vi "Terminal-Main-LoadingUnit.vi"(4 "ErrorQRef":refnum<queue>, 5 "ModbusNResRef":refnum<notifier>, 6 "ModbusMsgQRef":refnum<queue>, 7 "ModbusNReqRef":refnum<notifier>, 8 "error in (no error)":errorcluster caption="错误输入（无错误）", 11 "LoadingUnitNRef":refnum<notifier>) -> (0 "error out":errorcluster caption="错误输出")   [LabVIEW 2014]
panel:
  out "Loading Unit is running":bool
  out "LoadingUnit开始通知器":refnum<notifier>
  out "LoadingUnit开始响应器":refnum<notifier>
  out "LoadingUnit停止通知器":refnum<notifier>
  out "LoadingUnit停止响应器":refnum<notifier>
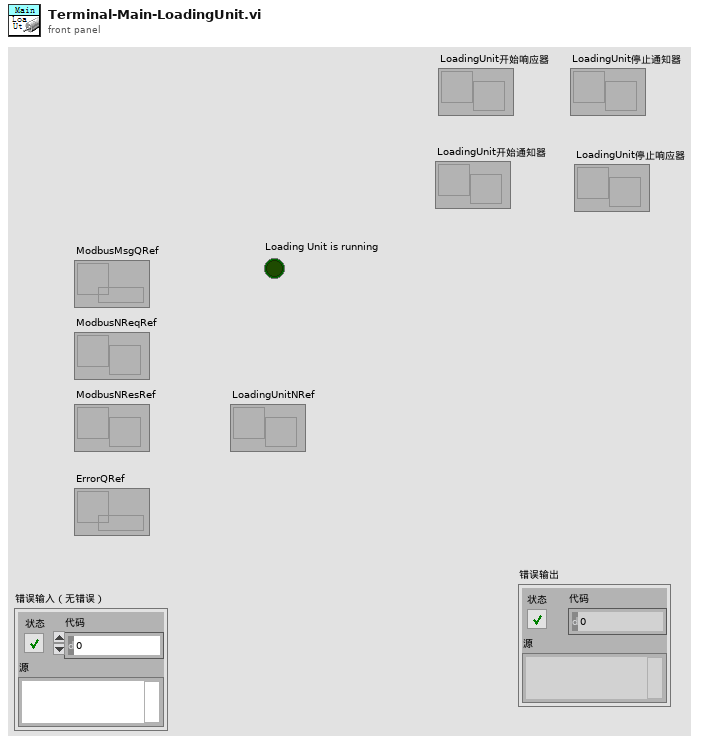
[diagram p1: front panel]
types:
  T1 = cluster{"Transaction ID":u16, "Unit ID":u8, "Starting Address":u16, "Quantity":u16}
  T2 = cluster{"Transaction ID":u16, "Unit ID":u8, "Address":u16, "Register":u16}
  T3 = cluster{"Transaction ID":u16, "Unit ID":u8, "Starting Address":u16, "Registers":u16[]}
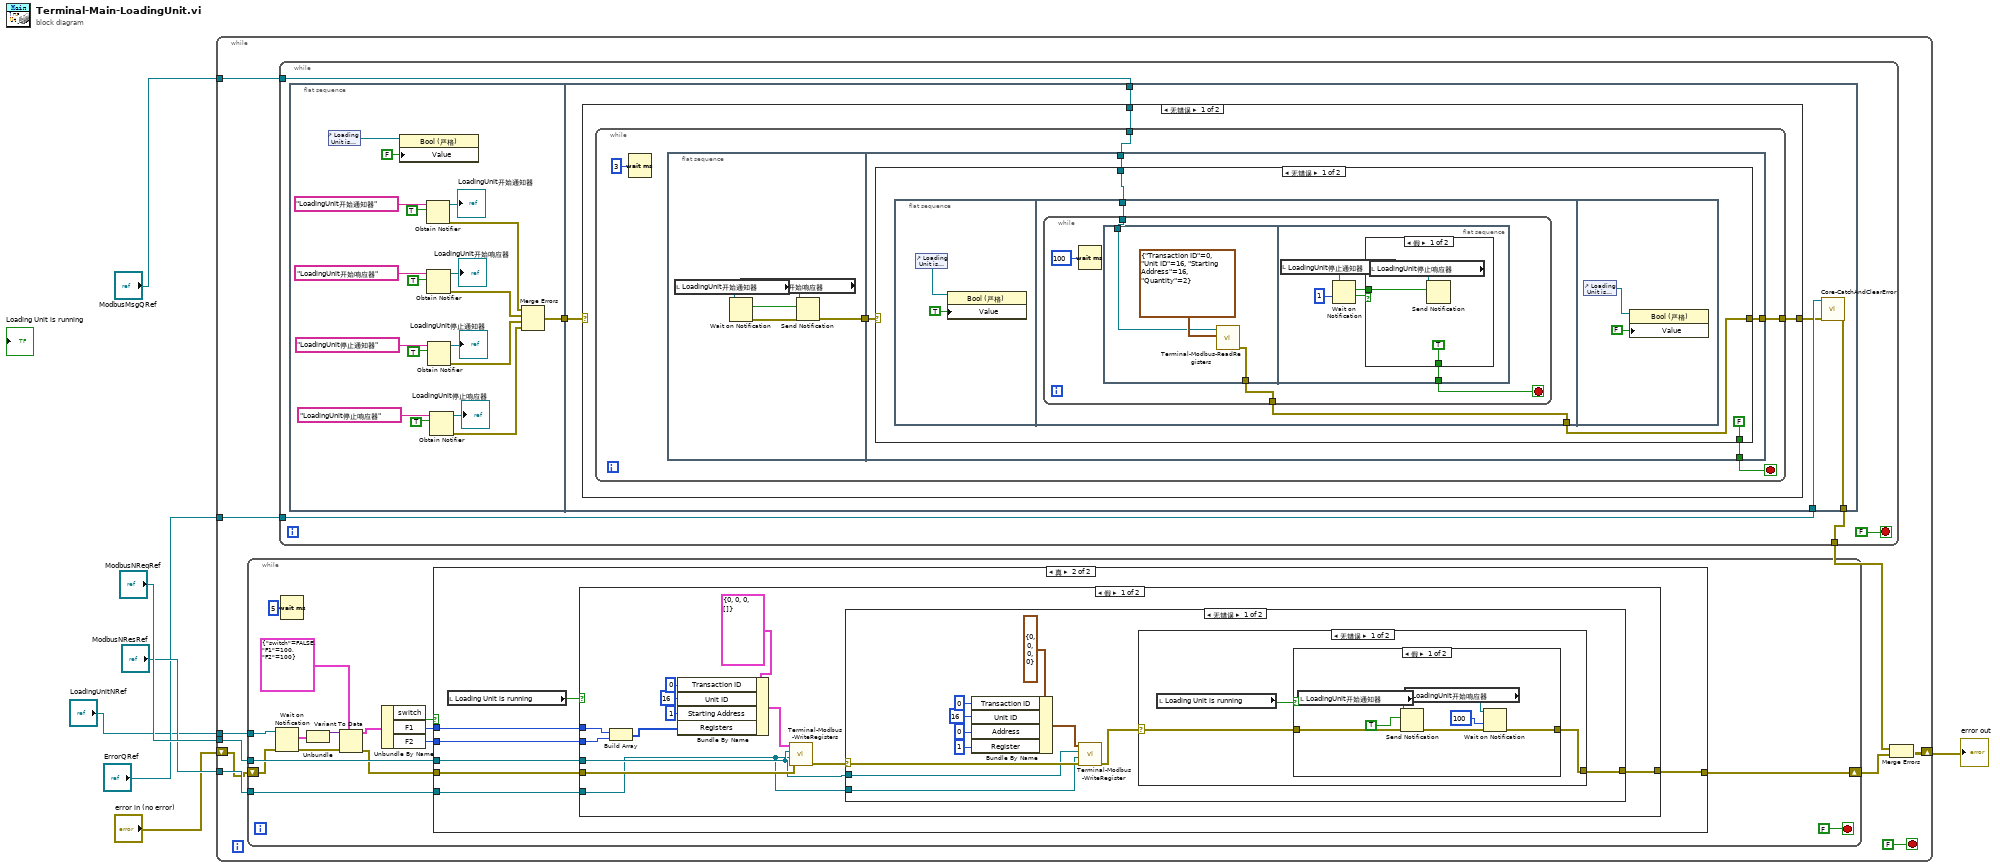
[diagram p0: block diagram]
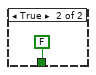
[diagram p2: hidden frame]
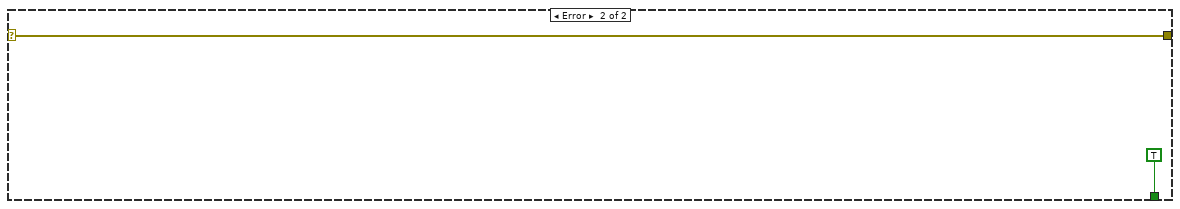
[diagram p3: hidden frame]
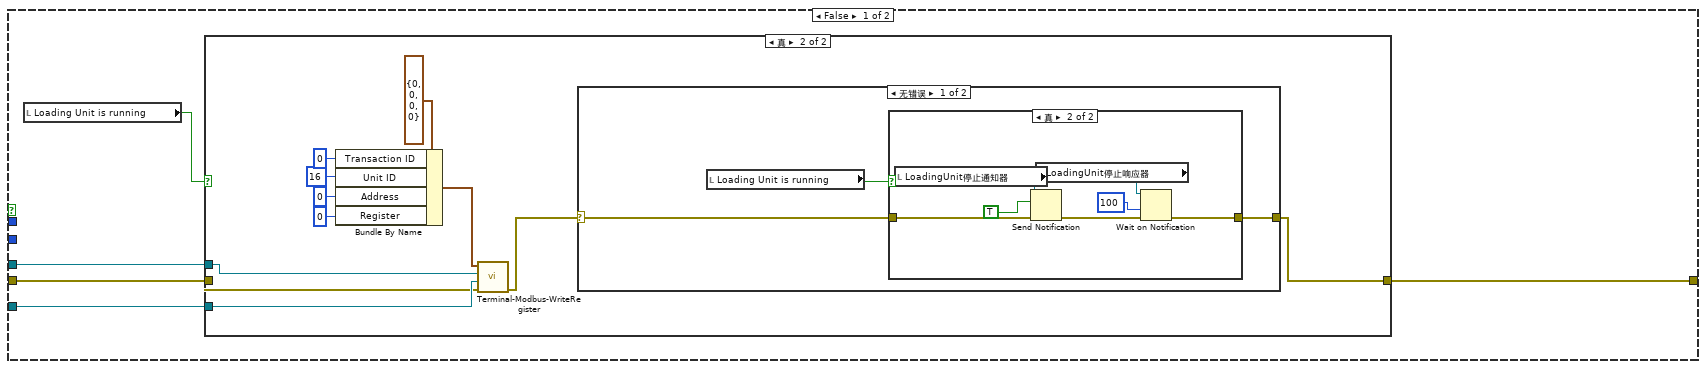
[diagram p5: hidden frame]
diagram:
  n1 = while {
    tunnel: "ModbusMsgQRef" -> [w17]
    tunnel: "ModbusNReqRef" -> [w16]
    tunnel: "ModbusNResRef" -> [w15]
    tunnel: "ErrorQRef" -> [w13]
    shift-right: [w12] -> w2
    shift-left: "error in (no error)" -> [w14]
    tunnel: "LoadingUnitNRef" -> [w8]
    stop <- FALSE stop-if-true
    n2 = while {
      tunnel: w16 -> [w106]
      tunnel: w15 -> [w105]
      shift-right: [w104] -> w11
      shift-left: w14 -> [w100]
      tunnel: w8 -> [w101]
      stop <- FALSE stop-if-true
      n3 = Wait on Notification(notifier=w101, error in (no error)=w100) -> (notification=w99:cluster{variant, string}, error out=w94:errorcluster)  [unwired: 2 in, 2 out]
      n4 = Wait (ms)(milliseconds to wait=u32 5 ("等待时间（毫秒）")) -> ()  [unwired: 1 out]
      n5 = Unbundle(w99) -> (w98:variant)  [unwired: 1 out]
      n6 = Variant To Data(error in=w94, type=cluster{"switch":bool, "F1":u16, "F2":u16} {"switch"=FALSE, "F1"=100, "F2"=100}, Variant=w98) -> (data=w97:cluster{"switch":bool, "F1":u16, "F2":u16}, error out=w93:errorcluster)
      n7 = Unbundle By Name(w97) -> ("switch"=w96:bool, "F1"=w95:u16, "F2"=w91:u16)
      n8 = case shown="真" w96 {
        tunnel: w106 -> [w111 w140]
        tunnel: w105 -> [w110 w141]
        tunnel: w93 -> [w109 w142]
        tunnel: [w108 w139] -> w104
        tunnel: w95 -> [_ w138]
        tunnel: w91 -> [_ w136]
        frame False {
          n9 = local read "Loading Unit is running"() -> (w107:bool)
          n10 = case shown="真" w107 {
            tunnel: w111 -> [_ w122]
            tunnel: w110 -> [_ w121]
            tunnel: w109 -> [w112 w120]
            tunnel: [w112 w119] -> w108
            frame False {
            }
            frame True {
              n11 = Bundle By Name(cluster=T2 {"Transaction ID"=0, "Unit ID"=0, "Address"=0, "Register"=0} ("簇"), "Transaction ID"=u16 0, "Unit ID"=u8 16, "Address"=u16 0, "Register"=u16 0) -> (w114:T2)
              n12 = call "Terminal-Modbus-WriteRegister.vi"("error in (no error)"=w120, "ModbusNResRef"=w121, "ModbusNReqRef"=w122, "簇"=w114) -> ("error out"=w123:errorcluster)  [unwired: 7 in]
              n13 = case shown="无错误" w123 {
                selector: w123 -> [w125 w135]
                tunnel: [w124 w135] -> w119
                frame No Error {
                  n14 = local read "Loading Unit is running"() -> (w126:bool)
                  n15 = case shown="真" w126 {
                    tunnel: [w127 w129] -> w124
                    tunnel: w125 -> [w127 w128]
                    frame False {
                    }
                    frame True {
                      n16 = local read "LoadingUnit停止通知器"() -> (w134:refnum<notifier>)
                      n17 = Send Notification(notification=TRUE ("通知"), notifier=w134, error in (no error)=w128) -> (error out=w132:errorcluster)  [unwired: 1 out]
                      n18 = local read "LoadingUnit停止响应器"() -> (w131:refnum<notifier>)
                      n19 = Wait on Notification(notifier=w131, timeout in ms (-1)=100 ("超时毫秒(-1)"), error in (no error)=w132) -> (error out=w129:errorcluster)  [unwired: 1 in, 3 out]
                    }
                  }
                }
                frame Error {
                }
              }
            }
          }
        }
        frame True {
          n20 = local read "Loading Unit is running"() -> (w137:bool)
          n21 = case shown="假" w137 {
            tunnel: w142 -> [w154 w180]
            tunnel: w141 -> [w143 _]
            tunnel: w140 -> [w144 _]
            tunnel: [w153 w180] -> w139
            tunnel: w138 -> [w152 _]
            tunnel: w136 -> [w151 _]
            frame False {
              n22 = Build Array(w152, w151) -> (w145:u16[])
              n23 = Bundle By Name(cluster=T3 {"Transaction ID"=0, "Unit ID"=0, "Starting Address"=0, "Registers"=[]} ("簇"), "Transaction ID"=u16 0, "Unit ID"=u8 16, "Starting Address"=u16 1 ("Address"), "Registers"=w145) -> (w147:T3)
              n24 = call "Terminal-Modbus-WriteRegisters.vi"("error in (no error)"=w154, "ModbusNResRef"=w143, "ModbusNReqRef"=w144, "簇"=w147) -> ("error out"=w155:errorcluster)  [unwired: 7 in]
              n25 = case shown="无错误" w155 {
                selector: w155 -> [w165 w179]
                tunnel: w144 -> [w164 _]
                tunnel: w143 -> [w163 _]
                tunnel: [w162 w179] -> w153
                frame No Error {
                  n26 = Bundle By Name(cluster=T2 {"Transaction ID"=0, "Unit ID"=0, "Address"=0, "Register"=0} ("簇"), "Transaction ID"=u16 0, "Unit ID"=u8 16, "Address"=u16 0, "Register"=u16 1) -> (w157:T2)
                  n27 = call "Terminal-Modbus-WriteRegister.vi"("error in (no error)"=w165, "ModbusNResRef"=w163, "ModbusNReqRef"=w164, "簇"=w157) -> ("error out"=w166:errorcluster)  [unwired: 7 in]
                  n28 = case shown="无错误" w166 {
                    selector: w166 -> [w168 w178]
                    tunnel: [w167 w178] -> w162
                    frame No Error {
                      n29 = local read "Loading Unit is running"() -> (w169:bool)
                      n30 = case shown="假" w169 {
                        tunnel: [w171 w177] -> w167
                        tunnel: w168 -> [w170 w177]
                        frame False {
                          n31 = local read "LoadingUnit开始通知器"() -> (w176:refnum<notifier>)
                          n32 = Send Notification(notification=TRUE ("通知"), notifier=w176, error in (no error)=w170) -> (error out=w174:errorcluster)  [unwired: 1 out]
                          n33 = local read "LoadingUnit开始响应器"() -> (w173:refnum<notifier>)
                          n34 = Wait on Notification(notifier=w173, timeout in ms (-1)=100 ("超时毫秒(-1)"), error in (no error)=w174) -> (error out=w171:errorcluster)  [unwired: 1 in, 3 out]
                        }
                        frame True {
                        }
                      }
                    }
                    frame Error {
                    }
                  }
                }
                frame Error {
                }
              }
            }
            frame True {
            }
          }
        }
      }
    }
    n35 = while {
      tunnel: w17 -> [w21]
      tunnel: w13 -> [w20]
      tunnel: [w18] -> w10
      stop <- FALSE stop-if-true
      n36 = flat-sequence {
        tunnel: [w24] -> w22
        tunnel: w22 -> [w46]
        tunnel: w20 -> [w45]
        tunnel: [w43] -> w18
        tunnel: w21 -> [w42]
        frame #0 {
          n37 = control-ref of="Loading Unit is running"() -> (w23:refnum<vi>)
          n38 = property class="Bool (严格)"(reference=w23, "Value"=FALSE ("值")) -> ()  [unwired: 1 in, 2 out]
          n39 = Obtain Notifier(name (unnamed)="LoadingUnit开始通知器" ("名称（未命名）"), notification data type=TRUE) -> (notifier out=→"LoadingUnit开始通知器":refnum<notifier>, error out=w28:errorcluster)  [unwired: 2 in, 1 out]
          n40 = Obtain Notifier(name (unnamed)="LoadingUnit开始响应器" ("名称（未命名）"), notification data type=TRUE) -> (notifier out=→"LoadingUnit开始响应器":refnum<notifier>, error out=w27:errorcluster)  [unwired: 2 in, 1 out]
          n41 = Obtain Notifier(name (unnamed)="LoadingUnit停止通知器" ("名称（未命名）"), notification data type=TRUE) -> (notifier out=→"LoadingUnit停止通知器":refnum<notifier>, error out=w26:errorcluster)  [unwired: 2 in, 1 out]
          n42 = Obtain Notifier(name (unnamed)="LoadingUnit停止响应器" ("名称（未命名）"), notification data type=TRUE) -> (notifier out=→"LoadingUnit停止响应器":refnum<notifier>, error out=w25:errorcluster)  [unwired: 2 in, 1 out]
          n43 = Merge Errors(w28, w27, w26, w25) -> (w24:errorcluster)
        }
        frame #1 {
          n44 = case shown="无错误" w46 {
            selector: w46 -> [_ w90]
            tunnel: [w48 w90] -> w44
            tunnel: w42 -> [w47 _]
            frame No Error {
              n45 = while {
                tunnel: [w51] -> w48
                tunnel: w47 -> [w50]
                stop <- w52 stop-if-true
                n46 = Wait (ms)(milliseconds to wait=u32 3 ("等待时间（毫秒）")) -> ()  [unwired: 1 out]
                n47 = flat-sequence {
                  tunnel: [w54] -> w53
                  tunnel: w53 -> [w62]
                  tunnel: [w61] -> w52
                  tunnel: [w60] -> w51
                  tunnel: w50 -> [w59]
                  frame #0 {
                    n48 = local read "LoadingUnit开始通知器"() -> (w58:refnum<notifier>)
                    n49 = Wait on Notification(notifier=w58) -> (notification=w55:bool, error out=w56:errorcluster)  [unwired: 3 in, 2 out]
                    n50 = local read "LoadingUnit开始响应器"() -> (w57:refnum<notifier>)
                    n51 = Send Notification(notification=w55, notifier=w57, error in (no error)=w56) -> (error out=w54:errorcluster)  [unwired: 1 out]
                  }
                  frame #1 {
                    n52 = case shown="无错误" w62 {
                      selector: w62 -> [_ w88]
                      tunnel: [FALSE TRUE] -> w61
                      tunnel: [w64 w88] -> w60
                      tunnel: w59 -> [w63 _]
                      frame No Error {
                        n53 = flat-sequence {
                          tunnel: [w68] -> w64
                          tunnel: w63 -> [w69]
                          frame #0 {
                            n54 = control-ref of="Loading Unit is running"() -> (w66:refnum<vi>)
                            n55 = property class="Bool (严格)"(reference=w66, "Value"=TRUE ("值")) -> ()  [unwired: 1 in, 2 out]
                          }
                          frame #1 {
                            n56 = while {
                              tunnel: w69 -> [w73]
                              tunnel: [w72] -> w68
                              stop <- w71 stop-if-true
                              n57 = Wait (ms)(milliseconds to wait=u32 100 ("等待时间（毫秒）")) -> ()  [unwired: 1 out]
                              n58 = flat-sequence {
                                tunnel: w73 -> [w75]
                                tunnel: [w74] -> w72
                                tunnel: [w77] -> w71
                                frame #0 {
                                n59 = call "Terminal-Modbus-ReadRegisters.vi"("簇"=T1 {"Transaction ID"=0, "Unit ID"=16, "Starting Address"=16, "Quantity"=2}, "ModbusMsgQRef"=w75) -> ("error out"=w74:errorcluster)  [unwired: 9 in]
                                }
                                frame #1 {
                                n60 = local read "LoadingUnit停止通知器"() -> (w80:refnum<notifier>)
                                n61 = Wait on Notification(notifier=w80, timeout in ms (-1)=1 ("超时毫秒(-1)")) -> (notification=w78:bool, timed out?=w79:bool)  [unwired: 2 in, 2 out]
                                n62 = case shown="假" w79 {
                                tunnel: [TRUE FALSE] -> w77
                                tunnel: w78 -> [w83 _]
                                frame False {
                                n63 = local read "LoadingUnit停止响应器"() -> (w82:refnum<notifier>)
                                n64 = Send Notification(notification=w83, notifier=w82) -> ()  [unwired: 1 in, 2 out]
                                }
                                frame True {
                                }
                                }
                                }
                              }
                            }
                          }
                          frame #2 {
                            n65 = control-ref of="Loading Unit is running"() -> (w86:refnum<vi>)
                            n66 = property class="Bool (严格)"(reference=w86, "Value"=FALSE ("值")) -> ()  [unwired: 1 in, 2 out]
                          }
                        }
                      }
                      frame Error {
                      }
                    }
                  }
                }
              }
            }
            frame Error {
            }
          }
          n67 = call "Core-CatchAndClearError.vi"("error in (no error)"=w44, "ErrorQ"=w45) -> ("error out"=w43:errorcluster)  [unwired: 7 in]
        }
      }
    }
    n68 = Merge Errors(w10, w11) -> (w12:errorcluster)
  }
  "error out" <- w2
